vi "Connect.vi"(8 "error in (no error)":errorcluster, 10 "COM Settings":T1={"baud rate"=9600, "data bits"=8, "parity"=enum."None", "stop bits"=10, "flow control"=0} {"flow control" items=["None"=0, "XON/XOFF"=1, "RTS/CTS"=2, "DTR/DSR"=4]; "stop bits" items=["1.0"=10, "1.5"=15, "2.0"=20]; "data bits" min=5 max=8 step=1; "baud rate" items=["75"=75, "110"=110, "134"=134, "150"=150, "300"=300, "600"=600, "1200"=1200, "1800"=1800, "2400"=2400, "4800"=4800, "7200"=7200, "9600"=9600, "14400"=14400, "19200"=19200, "28800"=28800, "38400"=38400, "56000"=56000, "57600"=57600, "115200"=115200, "128000"=128000, "230400"=230400]}, 11 "VISA resource name":refnum<visa-resource-name>) -> (0 "error out":errorcluster, 3 "VISA resource name out":refnum<visa-resource-name>)   [LabVIEW 2019, in "Mark 10 TSTM-DC.lvlib"]
uses:
  Mark 10 TSTM-DC.lvlib
  Cluster - COMSettings.ctl
  <vilib>/Instr/_visa.llb/VISA Configure Serial Port (Instr).vi
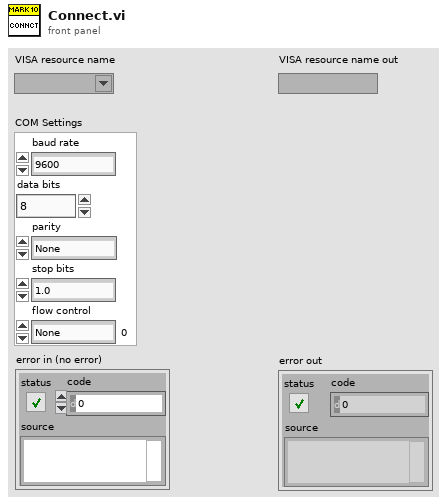
[diagram p1: front panel]
types:
  T1 = typedef "Mark 10 TSTM-DC.lvlib/Cluster - COMSettings.ctl" = cluster{"baud rate":u32, "data bits":u16, "parity":enum16{"None", "Odd", "Even", "Mark", "Space"}, "stop bits":u16, "flow control":u16}
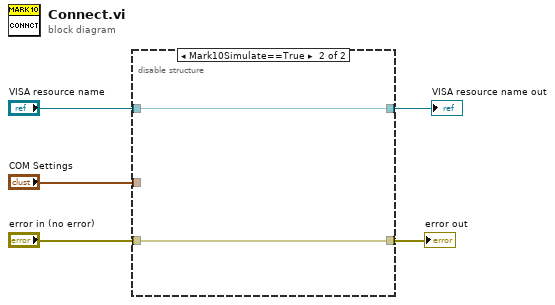
[diagram p0: block diagram]
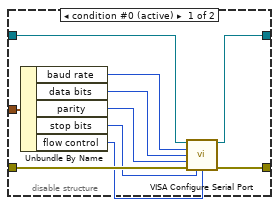
[diagram p2: hidden frame]
diagram:
  n1 = disable-structure shown="Mark10Simulate==True" {
    disable-tunnel: "error in (no error)" -> [w15 w16]
    disable-tunnel: [w14 w16] -> w4
    disable-tunnel: "COM Settings" -> [w13 _]
    disable-tunnel: "VISA resource name" -> [w7 w17]
    disable-tunnel: [w6 w17] -> w1
    frame condition #0 (active) {
      n2 = Unbundle By Name(w13) -> ("baud rate"=w8:u32, "data bits"=w9:u16, "parity"=w10:enum16{"None", "Odd", "Even", "Mark", "Space"}, "stop bits"=w11:u16, "flow control"=w12:u16)
      n3 = call-poly "VISA Configure Serial Port"("VISA resource name"=w7, "baud rate (9600)"=w8, "data bits (8)"=w9, "parity (0:none)"=w10, "error in (no error)"=w15, "stop bits (10: 1 bit)"=w11, "flow control (0:none)"=w12) -> ("VISA resource name out"=w6:refnum<visa-resource-name>, "error out"=w14:errorcluster)  [unwired: 7 in]
    }
    frame condition #1 {
    }
  }
  "error out" <- w4
  "VISA resource name out" <- w1
